vi "Create New File (no overwrite).vi"(8 "Error In":errorcluster, 9 "Dialog?":bool, 11 "New Path":path) -> (0 "Error Out":errorcluster, 3 "New (modified) Path":path)   [LabVIEW 2021, in "Files.lvlib"]
doc: "This VI checks that the provided path is not used.\nIf it is, it returns a path with a number suffix that is not used at that time."
uses:
  Files.lvlib
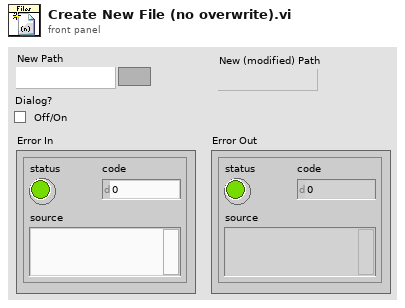
[diagram p1: front panel]
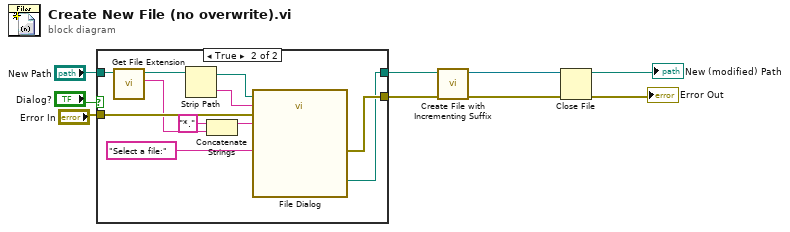
[diagram p0: block diagram]
diagram:
  n1 = case shown="True" "Dialog?" {
    tunnel: "New Path" -> [w11 w21]
    tunnel: [w11 w19] -> w3
    tunnel: "Error In" -> [w10 w22]
    tunnel: [w10 w20] -> w1
    frame False {
    }
    frame True {
      n2 = call <vilib>:"Get File Extension.vi"("file"=w21) -> ("lowercase file extension"=w14:string, "dup file"=w17:path)  [unwired: 6 in, 3 out]
      n3 = Strip Path(path=w17) -> (stripped path=w16:path, name=w15:string)
      n4 = Concatenate Strings("*." ("string"), w14) -> (w12:string)
      n5 = call "File Dialog"("start path"=w16, "prompt"="Select a file:", "default name"=w15, "error in"=w22, "pattern (all files)"=w12) -> ("selected path"=w19:path, "error out"=w20:errorcluster)  [unwired: 7 in, 2 out]
    }
  }
  n6 = call <vilib>:"Create File with Incrementing Suffix.vi"("error in (no error)"=w1, "file path"=w3) -> ("error out"=w8:errorcluster, "refnum out"=w9:refnum<file>)  [unwired: 7 in, 1 out]
  n7 = Close File(refnum=w9, error in=w8) -> (path=→"New (modified) Path":path, error out=→"Error Out":errorcluster)
